vi "StartTest_WithTestCase_AddsTestCase.vi"() -> ()   [LabVIEW 2017, in "ResultTreeListener.Tests.lvlib"]
uses:
  ResultTreeListener.Tests.lvlib
  b9be8222-4629-4de4-b646-ac532e0c1106.vi
  Support/FakeTestCase/FakeTestCase.lvclass
  C:/Users/de200256/Code/logmanoriginal/lvunit/Test/Test.lvclass
  Constraint/IsEqual/Create.vi
  ResultTreeListener/ResultTreeListener.lvclass
  Constraint/IsEqual/IsEqual.lvclass
  ResultTree/ResultTree.lvclass
panel:
  out "error out":errorcluster
  in  "Tree":string(tree)
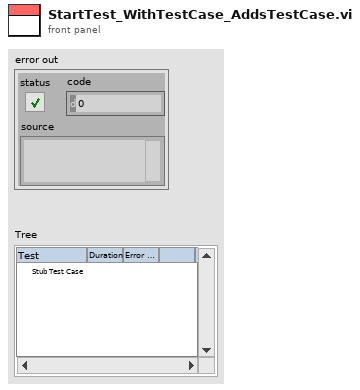
[diagram p1: front panel]
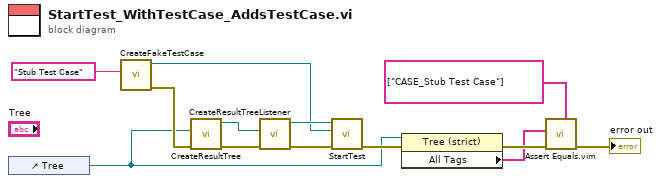
[diagram p0: block diagram]
diagram:
  n1 = control-ref of="Tree"() -> (w3:refnum<vi>)
  n2 = call "CreateFakeTestCase.vi"("Name"="Stub Test Case") -> ("error out"=w5:errorcluster, "FakeTestCase out"=w7:refnum<class "FakeTestCase.lvclass">)  [unwired: 9 in]
  n3 = call "CreateResultTree.vi"("error in (no error)"=w5, "Tree Refnum"=w3) -> ("error out"=w13:errorcluster, "ResultTree out"=w12:refnum<class "ResultTree.lvclass">)  [unwired: 8 in]
  n4 = call "CreateResultTreeListener.vi"("error in (no error)"=w13, "ResultTree"=w12) -> ("error out"=w11:errorcluster, "ResultTreeListener out"=w8:refnum<class "ResultTreeListener.lvclass">)  [unwired: 8 in]
  n5 = call-dynamic "StartTest.vi"("error in (no error)"=w11, "Test"=w7, "ResultTreeListener in"=w8) -> ("error out"=w9:errorcluster)  [unwired: 7 in, 1 out]
  n6 = property class="Tree (strict)"(reference=w3, error in=w9) -> (error out=w4:errorcluster, "All Tags"=w2:string[])  [unwired: 1 out]
  n7 = call "Assert Equals.vim"("Expected"=string[] ["CASE_Stub Test Case"] ("All Tags"), "error in (no error)"=w4, "Actual"=w2) -> ("error out"=→"error out":errorcluster)  [unwired: 8 in]
